vi "open.vi"(8 "error in (no error)":errorcluster caption="错误输入（无错误）", 11 "WebDAV client 输入":refnum<class "WebDAV client.lvclass">) -> (0 "error out":errorcluster caption="错误输出", 3 "WebDAV client 输出":refnum<class "WebDAV client.lvclass">)   [LabVIEW 2016, in "数据传输系统-04.lvlib" / "update.lvlib" / "WebDAV client.lvclass"]
uses:
  WebDAV client.lvclass
  WebDAV client.lvclass/WebDAV client.ctl
  <vilib>/WebDAVClient/NI_WebDAV.lvlib
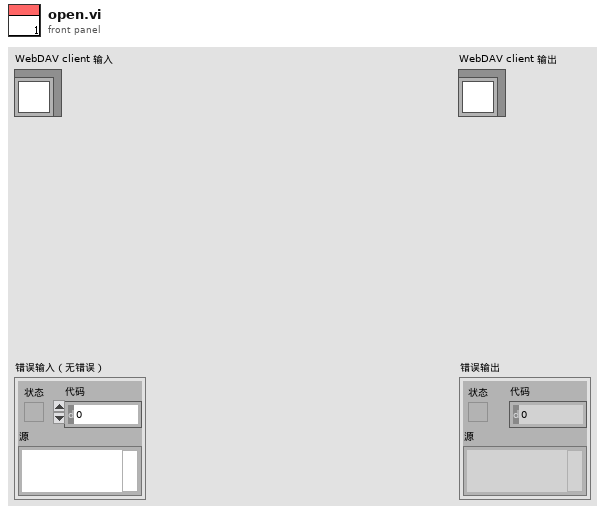
[diagram p1: front panel]
types:
  T1 = cluster{"URL":string, "USER":string, "PASSWORD":string}
  T2 = typedef "NI_WebDAV.lvlib/Asynchronous Session Handle.ctl" = refnum<k1>
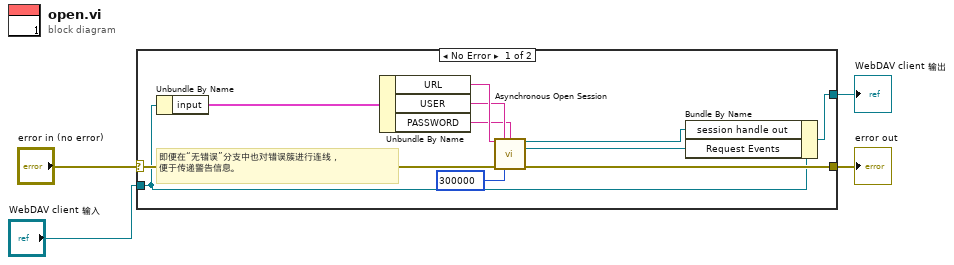
[diagram p0: block diagram]
diagram:
  n1 = case shown="No Error" "error in (no error)" {
    selector: "error in (no error)" -> [w12 w17]
    tunnel: [w11 w17] -> w3
    tunnel: [w9 w16] -> w1
    tunnel: "WebDAV client 输入" -> [w7 w16]
    frame No Error {
      # "即便在“无错误”分支中也对错误簇进行连线，\n便于传递警告信息。"
      n2 = Unbundle By Name(w7) -> ("input"=w6:T1)
      n3 = Unbundle By Name(w6) -> ("URL"=w15:string, "USER"=w14:string, "PASSWORD"=w13:string)
      n4 = call <vilib>:"Asynchronous Open Session.vi"("host uri prefix"=w15, "username"=w14, "password"=w13, "error in (no error)"=w12, "timeout ms"=300000) -> ("session handle out"=w10:T2, "Request Events"=w8:refnum<event-registration>, "error out"=w11:errorcluster)  [unwired: 8 in]
      n5 = Bundle By Name(cluster=w7, "session handle out"=w10, "Request Events"=w8) -> (w9:refnum<class "WebDAV client.lvclass">)
    }
    frame Error {
    }
  }
  "error out" <- w3
  "WebDAV client 输出" <- w1
